vi "picoharp_parse_records.vi"(8 "error in (no error)":errorcluster, 11 "hydraharp in":refnum<class "picoharp.lvclass">) -> (0 "error out":errorcluster, 3 "hydraharp out":refnum<class "picoharp.lvclass">)   [LabVIEW 2015, in "picoharp.lvclass"]
uses:
  picoharp.lvclass
  picoharp.lvclass/picoharp.ctl
  Hydraharp/hydraharp_panel/hpanel_acq_modes.ctl
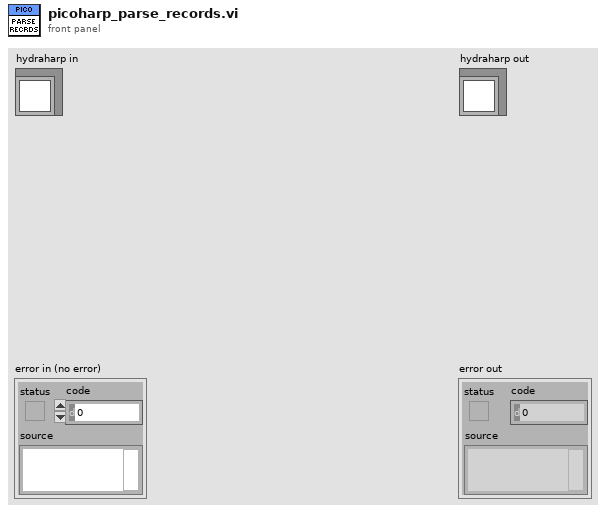
[diagram p1: front panel]
types:
  T1 = typedef "hpanel_acq_modes.ctl" = u16
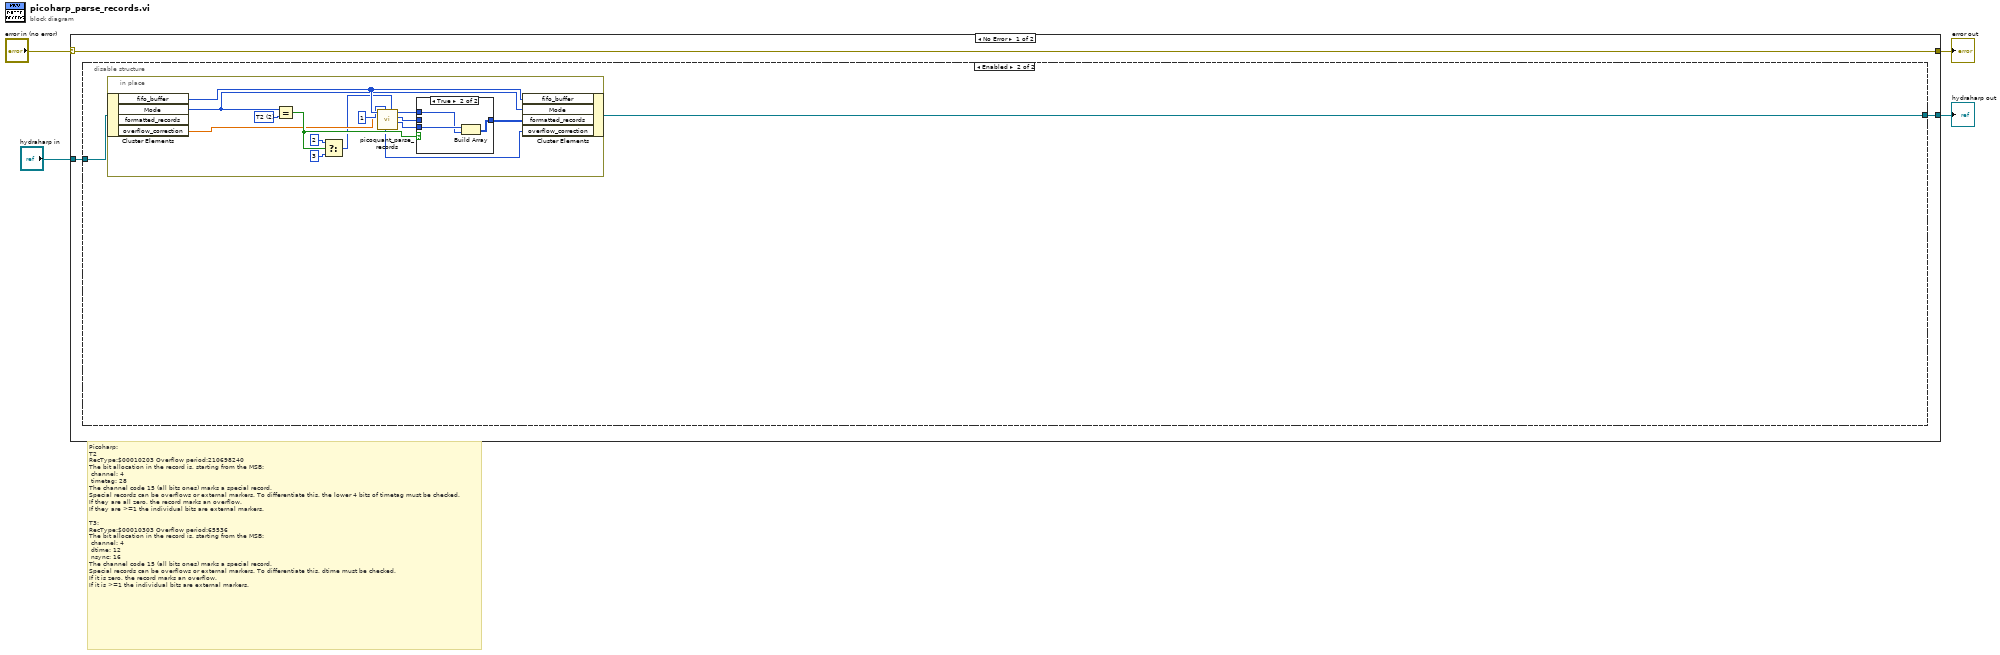
[diagram p0: block diagram]
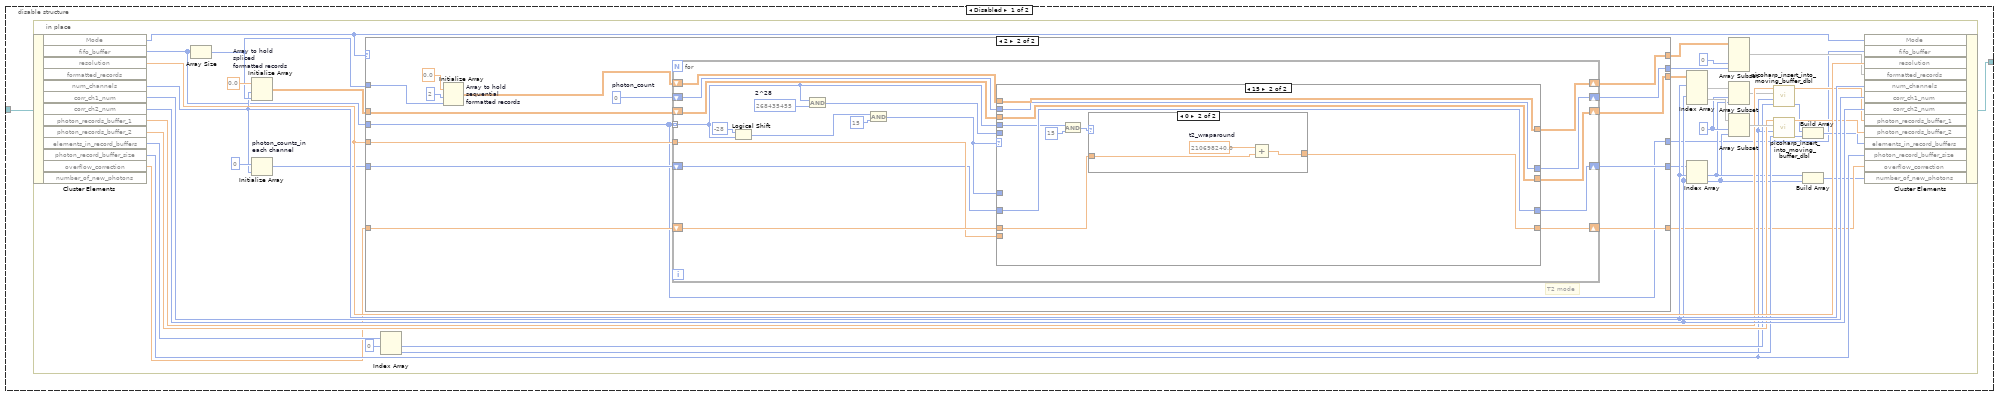
[diagram p2: hidden frame]
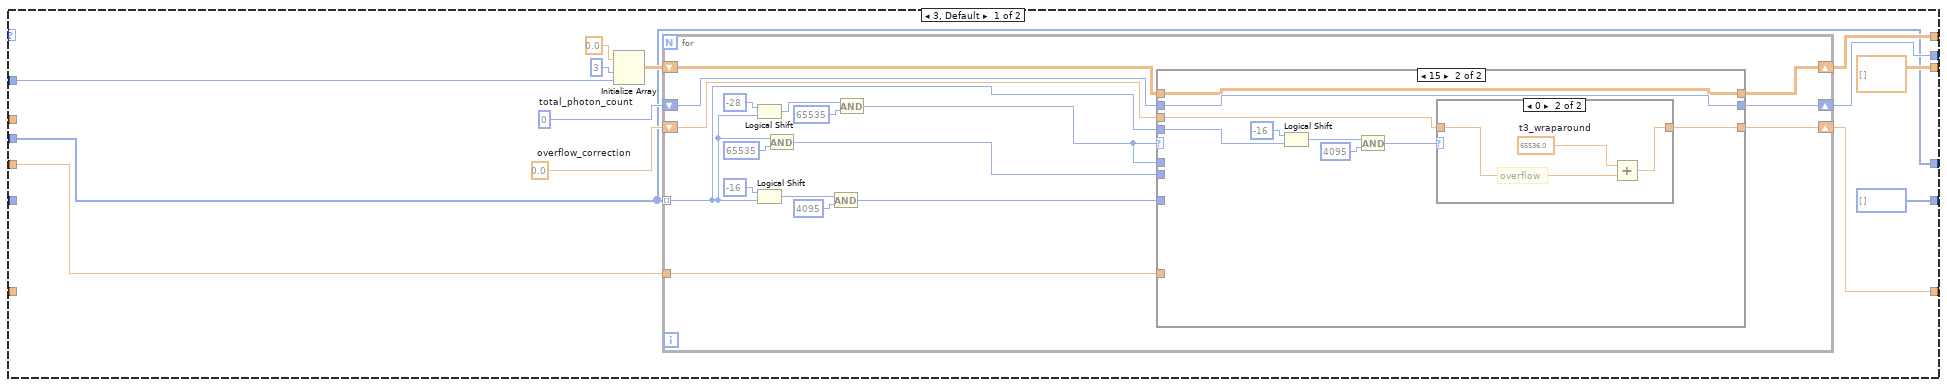
[diagram p3: hidden frame]
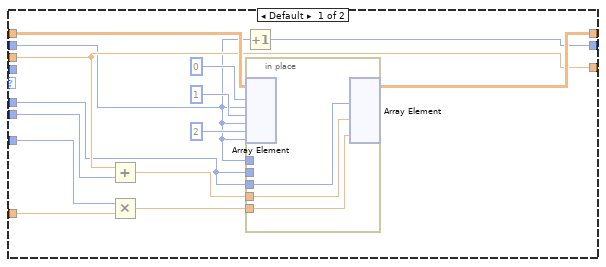
[diagram p4: hidden frame]
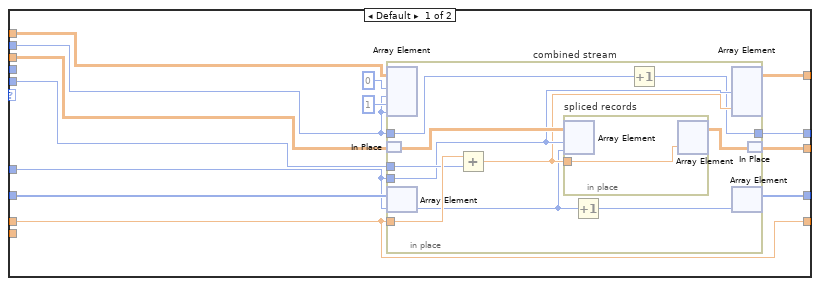
[diagram p6: hidden frame]
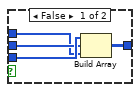
[diagram p8: hidden frame]
diagram:
  # "Picoharp:\nT2\nRecType:$00010203 Overflow period:210698240\nThe bit allocation in the record is, starting from the MSB:\n channel: 4\n timetag: 28\nThe channel code 15 (all bits ones) marks a special record.\nSpecial records can be overflows or external markers. To differentiate this, the lower 4 bits of timetag must be checked.\nIf they are all zero, the record marks an overflow.\nIf they are >=1 the individual bits are external markers.  \n\nT3:\nRecType:$00010303 Overflow period:65536\nThe bit allocation in the record is, starting from the MSB:\n channel: 4\n dtime: 12\n nsync: 16\nThe channel code 15 (all bits ones) marks a special record.\nSpecial records can be overflows or external markers. To differentiate this, dtime must be checked.\nIf it is zero, the record marks an overflow.\nIf it is >=1 the individual bits are external markers."
  n1 = case shown="No Error" "error in (no error)" {
    selector: "error in (no error)" -> [w7 w205]
    tunnel: [w7 w205] -> w3
    tunnel: [w5 w204] -> w1
    tunnel: "hydraharp in" -> [w6 w204]
    frame No Error {
      n2 = disable-structure shown="Enabled" {
        disable-tunnel: w6 -> [w9 w182]
        disable-tunnel: [w8 w181] -> w5
        frame Disabled {
          n3 = in-place {
            w34 = 0 ("index")
            n4 = in-place-cluster #1(w9) -> ("Mode"=w49:T1, "fifo_buffer"=w18:u32[], "resolution"=w48:dbl, "num_channels"=w39:i32, "corr_ch1_num"=w32:i32, "corr_ch2_num"=w31:i32, "photon_records_buffer_1"=w30:dbl[], "photon_records_buffer_2"=w29:dbl[], "elements_in_record_buffers"=w26:i32[], "photon_record_buffer_size"=w19:i32, "overflow_correction"=w17:dbl)  [unwired: 2 out]
            n5 = Array Size(array=w18) -> (size(s)=w42:i32)
            n6 = Initialize Array "Array to hold\nspliced\nformatted records"(0.0 ("element"), w39, w42) -> (w41:dbl[][])
            n7 = Initialize Array "photon_counts_in\neach channel"(0 ("element"), w39) -> (w38:i32[])
            n8 = case shown="2" w49 {
              tunnel: w18 -> [w50 w111]
              tunnel: w48 -> [w57 w122]
              tunnel: [w56 w121] -> w47
              tunnel: [w55 w120] -> w46
              tunnel: w42 -> [w54 w118]
              tunnel: w41 -> [_ w117]
              tunnel: w38 -> [_ w116]
              tunnel: [dbl[][] [] w115] -> w37
              tunnel: [i32[] [] w114] -> w15
              tunnel: w17 -> [_ w113]
              tunnel: [w51 w112] -> w16
              tunnel: [w50 w111] -> w10
              frame 3, Default {
                w58 = 0  # total_photon_count
                w59 = 0.0  # overflow_correction
                n9 = Initialize Array(0.0 ("element"), 3 ("dimension size"), w54) -> (w60:dbl[][])
                n10 = for {
                  tunnel: w50 -> [w63] mode=indexing
                  shift-right: [w67] -> w56
                  shift-left: w60 -> [w73]
                  shift-right: [w65] -> w51
                  shift-left: w59 -> [w72]
                  tunnel: w57 -> [w69]
                  shift-right: [w66] -> w55
                  shift-left: w58 -> [w68]
                  n11 = Logical Shift(y=i16 -28, x=w63) -> (x << y=w75:u32)
                  n12 = Logical Shift(y=i16 -16, x=w63) -> (x << y=w78:u32)
                  n13 = And(x=w63, y=u32 65535) -> (x .and. y?=w71:u32)
                  n14 = And(x=w78, y=u32 4095) -> (x .and. y?=w70:u32)
                  n15 = And(x=w75, y=u32 65535) -> (x .and. y?=w64:u32)
                  n16 = case shown="15" w64 {
                    tunnel: w73 -> [w91 w103]
                    tunnel: w72 -> [w83 w106]
                    tunnel: w71 -> [w94 _]
                    tunnel: w70 -> [w92 _]
                    tunnel: w69 -> [w93 _]
                    tunnel: w64 -> [w82 _]
                    tunnel: w68 -> [w81 w104]
                    tunnel: [w85 w103] -> w67
                    tunnel: [w84 w104] -> w66
                    tunnel: [w83 w105] -> w65
                    tunnel: w63 -> [_ w98]
                    frame Default {
                      n17 = Add(x=w83, y=w94) -> (x+y=w87:dbl)
                      n18 = Multiply(x=w92, y=w93) -> (x*y=w86:dbl)
                      n19 = Increment(x=w81) -> (x+1=w84:i32)
                      n20 = in-place {
                        in-place-border: w82 -> [w97]
                        in-place-border: w87 -> [w96]
                        in-place-border: w86 -> [w95]
                        in-place-border: w82 -> [_]
                        in-place-border: w81 -> [_]
                        n21 = in-place-array #2(w91, 0, w81, 1, w81, 2, w81) -> ()  [unwired: 3 out]
                        n22 = in-place-array #2(w97, w96, w95) -> (w85:dbl[][])  [unwired: 6 out]
                      }
                    }
                    frame 15 {
                      n23 = Logical Shift(y=i16 -16, x=w98) -> (x << y=w101:u32)
                      n24 = And(x=w101, y=u32 4095) -> (x .and. y?=w99:u32)
                      n25 = case shown="0" w99 {
                        tunnel: w106 -> [w107 w110]
                        tunnel: [w107 w109] -> w105
                        frame Default {
                          # "markers"
                        }
                        frame 0 {
                          w108 = 65536.0  # t3_wraparound
                          # "overflow"
                          n26 = Add(x=w108, y=w110) -> (x+y=w109:dbl)
                        }
                      }
                    }
                  }
                }
              }
              frame 2 {
                w123 = 0  # photon_count
                # "T2 mode"
                n27 = Initialize Array "Array to hold\nsequential\nformatted records"(0.0 ("element"), 2 ("dimension size"), w118) -> (w119:dbl[][])
                n28 = for {
                  tunnel: w111 -> [w126] mode=indexing
                  shift-right: [w134] -> w121
                  shift-left: w119 -> [w139]
                  shift-right: [w133] -> w112
                  shift-left: w113 -> [w138]
                  tunnel: w122 -> [w136]
                  shift-right: [w128] -> w120
                  shift-left: w123 -> [w135]
                  shift-right: [w131] -> w115
                  shift-left: w117 -> [w132]
                  shift-right: [w129] -> w114
                  shift-left: w116 -> [w130]
                  w143 = u32 268435455  # 2^28
                  n29 = Logical Shift(y=i16 -28, x=w126) -> (x << y=w141:u32)
                  n30 = And(x=w126, y=w143) -> (x .and. y?=w137:u32)
                  n31 = And(x=w141, y=u32 15) -> (x .and. y?=w127:u32)
                  n32 = case shown="15" w127 {
                    tunnel: w139 -> [w156 w174]
                    tunnel: w138 -> [w152 w176]
                    tunnel: w137 -> [w151 _]
                    tunnel: w136 -> [_ _]
                    tunnel: w127 -> [w147 _]
                    tunnel: w135 -> [w145 w173]
                    tunnel: [w153 w174] -> w134
                    tunnel: [w152 w175] -> w133
                    tunnel: w132 -> [w150 w171]
                    tunnel: [w149 w171] -> w131
                    tunnel: w130 -> [w148 w172]
                    tunnel: [w146 w172] -> w129
                    tunnel: [w144 w173] -> w128
                    tunnel: w126 -> [_ w170]
                    frame Default {
                      n33 = in-place "combined stream" {
                        in-place-border: w147 -> [w163]
                        in-place-border: w152 -> [w166]
                        in-place-border: w151 -> [w165]
                        in-place-border: w145 -> [w158]
                        in-place-border: [w157] -> w144
                        n34 = in-place-array #3(w156, 0, w145, 1, w145) -> ()  [unwired: 2 out]
                        n35 = in-place-match #4(w150) -> (w164:dbl[][])
                        n36 = in-place-array #5(w148, w147) -> (w160:i32)
                        n37 = Add(x=w166, y=w165) -> (x+y=w161:dbl)
                        n38 = in-place "spliced records" {
                          in-place-border: w161 -> [w167]
                          n39 = in-place-array #6(w164, w163, w160) -> ()  [unwired: 1 out]
                          n40 = in-place-array #6(w167) -> (w162:dbl[][])  [unwired: 2 out]
                        }
                        n41 = Increment(x=w160) -> (x+1=w159:i32)
                        n42 = Increment(x=w158) -> (x+1=w157:i32)
                        n43 = in-place-array #3(w163, w161) -> (w153:dbl[][])  [unwired: 4 out]
                        n44 = in-place-array #5(w159) -> (w146:i32[])  [unwired: 1 out]
                        n45 = in-place-match #4(w162) -> (w149:dbl[][])
                      }
                    }
                    frame 15 {
                      n46 = And(x=w170, y=u32 15) -> (x .and. y?=w168:u32)
                      n47 = case shown="0" w168 {
                        tunnel: w176 -> [w177 w180]
                        tunnel: [w177 w179] -> w175
                        frame Default {
                          # "markers..."
                        }
                        frame 0 {
                          w178 = 210698240.0  # t2_wraparound
                          n48 = Add(x=w178, y=w180) -> (x+y=w179:dbl)
                        }
                      }
                    }
                  }
                }
              }
            }
            n49 = Index Array(array=w26, index #1=0 ("index")) -> (element #1=w24:i32, element #2=w23:i32)  [unwired: 1 in]
            n50 = Index Array(array=w37, index (row) #1=w32, index (row) #2=w31) -> (element #1=w36:dbl[], element #2=w35:dbl[])  [unwired: 2 in]
            n51 = Index Array(array=w15, index #1=w32, index #2=w31) -> (element #1=w14:i32, element #2=w13:i32)
            n52 = Array Subset(array=w47, index (col)=0 ("index"), length (col)=w46) -> (w44:dbl[][])  [unwired: 2 in]
            n53 = Array Subset(array=w36, index=w34, length=w14) -> (w11:dbl[])
            n54 = Array Subset(array=w35, index=w34, length=w13) -> (w33:dbl[])
            n55 = call "picoharp_insert_into_moving_buffer_dbl.vi"("elements_in_buffer"=w24, "buffer_size"=w19, "new_data"=w11, "buffer"=w30) -> ("elements_in_new_buffer"=w22:i32, "new_buffer"=w28:dbl[])  [unwired: 5 in, 1 out]
            n56 = call "picoharp_insert_into_moving_buffer_dbl.vi"("elements_in_buffer"=w23, "buffer_size"=w19, "new_data"=w33, "buffer"=w29) -> ("elements_in_new_buffer"=w21:i32, "new_buffer"=w27:dbl[])  [unwired: 5 in, 1 out]
            n57 = Build Array(w22, w21) -> (w20:i32[])
            n58 = Build Array(w14, w13) -> (w12:i32[])
            n59 = in-place-cluster #1("Mode"=w49, "fifo_buffer"=w10, "resolution"=w48, "formatted_records"=w44, "num_channels"=w39, "corr_ch1_num"=w32, "corr_ch2_num"=w31, "photon_records_buffer_1"=w28, "photon_records_buffer_2"=w27, "elements_in_record_buffers"=w20, "photon_record_buffer_size"=w19, "overflow_correction"=w16, "number_of_new_photons"=w12) -> (w8:refnum<class "picoharp.lvclass">)
          }
        }
        frame Enabled {
          n60 = in-place {
            w196 = T1 2 items=["T2"=2, "T3"=3] ("Mode")
            n61 = in-place-cluster #7(w182) -> ("fifo_buffer"=w190:u32[], "Mode"=w189:T1, "overflow_correction"=w184:dbl)  [unwired: 1 out]
            n62 = Equal?(x=w189, y=w196) -> (x = y?=w187:bool)
            n63 = Select(t=u8 2 ("tmode"), s=w187, f=u8 3) -> (s? t:f=w183:u8)
            n64 = call "picoquant_parse_records.vi"("acq_mode"=w183, "Device"=u8 1 ("device"), "overflow"=w184, "fifo_buffer"=w190) -> ("sync"=w193:u64[], "channels"=w192:u8[], "times"=w191:u64[], "overflow"=w186:u64)  [unwired: 2 in, 2 out]
            n65 = case shown="True" w187 {
              tunnel: w193 -> [w200 w203]
              tunnel: w192 -> [w199 _]
              tunnel: w191 -> [w198 w202]
              tunnel: [w197 w201] -> w188
              frame False {
                n66 = Build Array(w200, w199, w198) -> (w197:u64[][])
              }
              frame True {
                n67 = Build Array(w203, w202) -> (w201:u64[][])
              }
            }
            n68 = in-place-cluster #7("fifo_buffer"=w190, "Mode"=w189, "formatted_records"=w188, "overflow_correction"=w186) -> (w181:refnum<class "picoharp.lvclass">)
          }
        }
      }
    }
    frame Error {
    }
  }
  "error out" <- w3
  "hydraharp out" <- w1
